vi "Get Enqueuer ID.vi"(11 "Message Enqueuer in":refnum<class "Message Enqueuer.lvclass">) -> (2 "Valid Enqueuer?":bool, 3 "Enqueuer ID string out":string)   [LabVIEW 2020]
doc: "Get the unique ID from 'Message Enqueuer'."
uses:
  PPL/HDH.Actor Framework.Core.Actor.lvlibp/1abvi3w/vi.lib/ActorFramework/Message Enqueuer/Message Enqueuer.lvclass
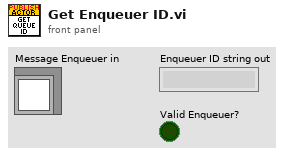
[diagram p1: front panel]
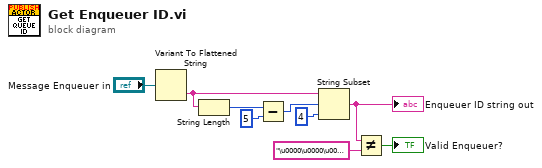
[diagram p0: block diagram]
diagram:
  n1 = Variant To Flattened String(Variant="Message Enqueuer in") -> (data string=w8:string)  [unwired: 1 out]
  n2 = String Length(string=w8) -> (length=w5:i32)
  n3 = Subtract(x=w5, y=5) -> (x-y=w7:i32)
  n4 = String Subset(string=w8, offset (0)=w7, length (rest)=4 ("length (rest)")) -> (substring=w3:string)
  "Enqueuer ID string out" <- w3
  n5 = Not Equal?(x=w3, y="\u0000\u0000\u0000\u0000") -> (x != y?=→"Valid Enqueuer?":bool)
